vi "_Destroy.vi"(8 "error in (no error)":errorcluster, 11 "Analog Output in":refnum<class "Analog Output.lvclass">) -> (0 "error out":errorcluster)   [LabVIEW 2017, in "Analog Output.lvclass"]
doc: "Superclass destructor: close all handles to and release all resources associated with this Instrument, then deallocate it. \n\nIMPORTANT: when destroying a class that inherits from Instrument, destroy your subclass first, and call the parent Instrument::_Destroy.vi LAST. This ensures your subclass destructor operates on a valid Instrument while it releases its resources."
uses:
  Analog Output.lvclass
  Analog Output.lvclass/Analog Output.ctl
  Utility Classes/Scannable/Scannable.lvclass
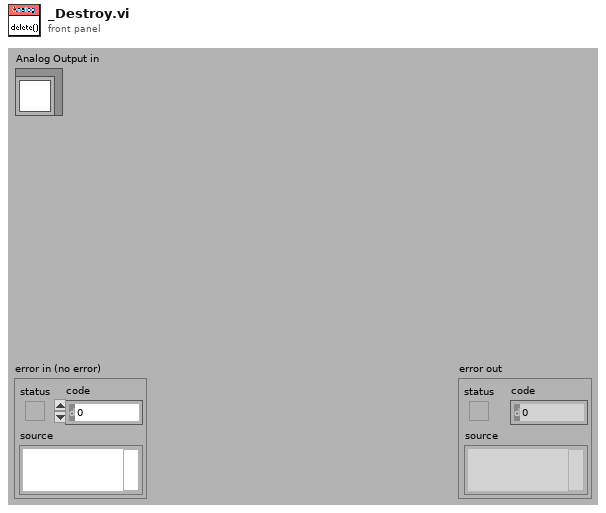
[diagram p1: front panel]
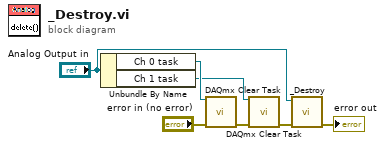
[diagram p0: block diagram]
diagram:
  n1 = Unbundle By Name("Analog Output in") -> ("Ch 0 task"=w5:refnum<k21>, "Ch 1 task"=w4:refnum<k21>)
  n2 = call <vilib>:"DAQmx Clear Task.vi"("task in"=w5, "error in"="error in (no error)") -> ("error out"=w3:errorcluster)  [unwired: 13 in]
  n3 = call <vilib>:"DAQmx Clear Task.vi"("task in"=w4, "error in"=w3) -> ("error out"=w1:errorcluster)  [unwired: 13 in]
  n4 = call-parent "_Destroy.vi"("error in (no error)"=w1, "Instrument in"="Analog Output in") -> ("error out"=→"error out":errorcluster)  [unwired: 9 in]
